vi "SV Peak Levels (1 Ch) (SGL).vi"(7 "reset":bool, 11 "input signal":waveform(sgl)={"t0"=timestamp(0 s since 1904-01-01), "dt"=0.0, "Y"=[]}) -> (0 "minimum":sgl=nan, 1 "maximum":sgl=nan, 2 "max-min":sgl=nan, 3 "peak":sgl=nan, 4 "duration (s)":dbl, 5 "timestamp":timestamp)   [LabVIEW 2017]
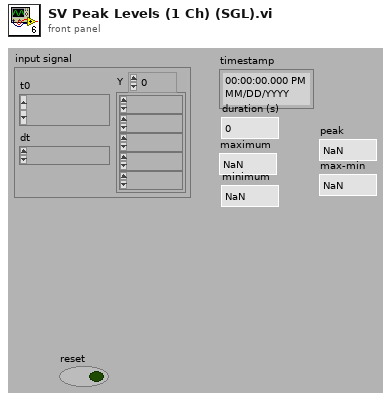
[diagram p1: front panel]
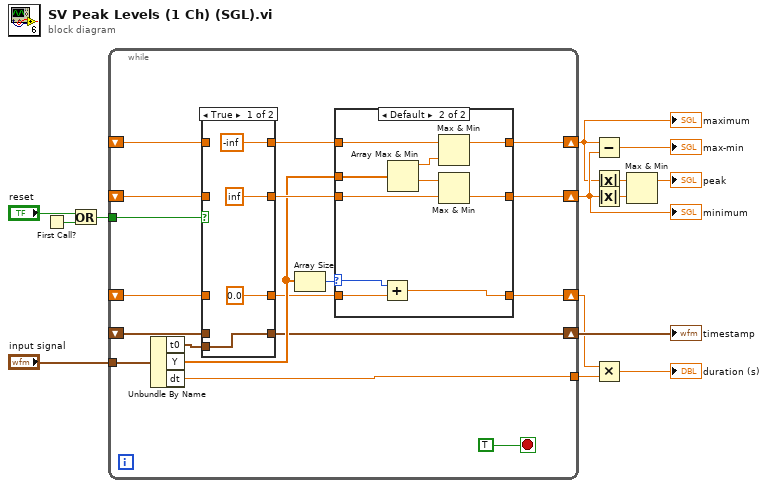
[diagram p0: block diagram]
diagram:
  n1 = First Call?() -> (First Call?: T/F=w5:bool)
  n2 = Or(x="reset", y=w5) -> (x .or. y?=w3:bool)
  n3 = while {
    tunnel: w3 -> [w22]
    shift-right: [w31] -> w1
    shift-left: _ -> [w25]
    shift-right: [w32] -> w2
    shift-left: _ -> [w26]
    shift-right: [w30] -> w7
    shift-left: _ -> [w15]
    tunnel: "input signal" -> [w29]
    shift-right: [w18] -> w9
    shift-left: _ -> [w19]
    tunnel: [w17] -> w8
    stop <- TRUE stop-if-true
    n4 = Unbundle By Name(w29) -> ("t0"=w20:timestamp, "Y"=w21:sgl[], "dt"=w17:dbl)
    n5 = case shown="True" w22 {
      tunnel: w26 -> [_ w39]
      tunnel: w25 -> [_ w40]
      tunnel: [sgl -inf ("t") w40] -> w24
      tunnel: [sgl inf ("t") w39] -> w23
      tunnel: w20 -> [w34 _]
      tunnel: w19 -> [_ w38]
      tunnel: [w34 w38] -> w18
      tunnel: [0.0 w37] -> w16
      tunnel: w15 -> [_ w37]
      frame True {
      }
      frame False {
      }
    }
    n6 = Array Size(array=w21) -> (size(s)=w28:i32)
    n7 = case shown="Default" w28 {
      selector: w28 -> [_ w49]
      tunnel: w24 -> [w43 w48]
      tunnel: w23 -> [w42 w47]
      tunnel: [w42 w53] -> w32
      tunnel: [w43 w52] -> w31
      tunnel: [w41 w51] -> w30
      tunnel: w16 -> [w41 w50]
      tunnel: w21 -> [_ w46]
      frame 0 {
      }
      frame Default {
        n8 = Add(x=w49, y=w50) -> (x+y=w51:dbl)
        n9 = Array Max & Min(array=w46) -> (max value=w45:sgl, min value=w44:sgl)  [unwired: 2 out]
        n10 = Max & Min(x=w48, y=w45) -> (max(x,y)=w52:sgl)  [unwired: 1 out]
        n11 = Max & Min(x=w44, y=w47) -> (min(x,y)=w53:sgl)  [unwired: 1 out]
      }
    }
  }
  "timestamp" <- w9
  "maximum" <- w1
  "minimum" <- w2
  n12 = Subtract(x=w1, y=w2) -> (x-y=→"max-min":sgl)
  n13 = Absolute Value(x=w1) -> (abs(x)=w13:sgl)
  n14 = Absolute Value(x=w2) -> (abs(x)=w12:sgl)
  n15 = Multiply(x=w7, y=w8) -> (x*y=→"duration (s)":dbl)
  n16 = Max & Min(x=w13, y=w12) -> (max(x,y)=→"peak":sgl)  [unwired: 1 out]
